vi "get_transitionTrigger.vi"(0 "NInstrSim_DFSMVisitor":refnum<class "NInstrSim_DFSMVisitor.lvclass">, 5 "error in (no error)":errorcluster) -> (14 "NInstrSim_DFSMVisitor":refnum<class "NInstrSim_DFSMVisitor.lvclass">, 16 "Trigger":T1, 17 "deviceVisitor":refnum<class "HGF_DeviceVisitor.lvclass">, 19 "error out":errorcluster)   [LabVIEW 2009, in "HGF_DIM_DFSM_Examples.lvlib" / "NInstrSim_DFSMVisitor.lvclass"]
doc: "This VI returns the HGF_DeviceFSM.lvsc transition trigger and device visitor."
uses:
  NInstrSim_DFSMVisitor.lvclass
  lib.lib/HGF_LVC/HGF_StateCharts/HGF_DeviceFSM/HGF_DeviceFSM.lvsc/Trigger.ctl
  lib.lib/HGF_LVC/HGF_DeviceBaseClasses/HGF_DeviceVisitor/HGF_DeviceVisitor.lvclass
  NInstrSim_ConfigureWaveformType/NInstrSim_ConfigureWaveformType.lvclass
  lib.lib/HGF_LVC/HGF_StateCharts/HGF_DFSMVisitor/HGF_DFSMVisitor.lvclass
  lib.lib/HGF_LVC/HGF_BaseClasses/HGF_NetworkVisitor/HGF_NetworkVisitor.lvclass
  lib.lib/HGF_LVC/HGF_StateCharts/HGF_DeviceFSM/HGF_DeviceFSM.lvsc
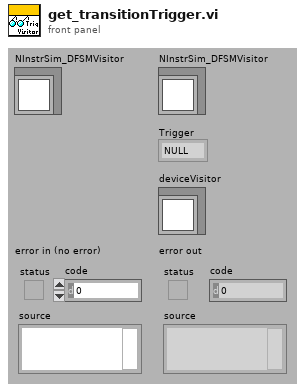
[diagram p1: front panel]
types:
  T1 = typedef "HGF_DeviceFSM.lvlib/HGF_DeviceFSM.lvsc/Trigger.ctl" = enum16{"NULL", "configure", "fault", "error", "resetError", "STOP", "visit", "not_configured", "done", "ok", "previsit", "configured"}
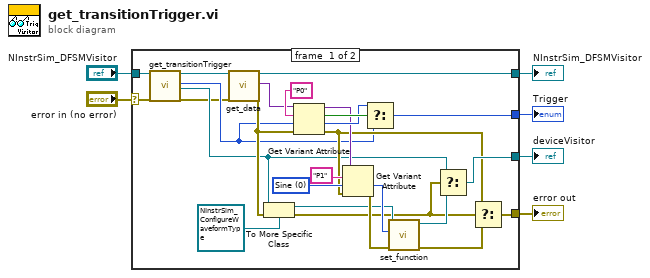
[diagram p0: block diagram]
diagram:
  n1 = case shown="No Error" "error in (no error)" {
    selector: "error in (no error)" -> [w7 w33]
    tunnel: [w13 w33] -> w1
    tunnel: [w30 w34] -> w4
    tunnel: "NInstrSim_DFSMVisitor" -> [w12 w34]
    tunnel: [w27 _] -> w3
    tunnel: [w24 _] -> w2
    frame #0 {
      w21 = u16 0 items=["Sine", "Square", "Sine+Noise", "Random", "Chirp"] ("function (0:Sine)")
      n2 = call-parent "get_transitionTrigger.vi"("HGF_DFSMVisitor"=w12, "error in (no error)"=w7) -> ("HGF_DFSMVisitor"=w11:refnum<class "NInstrSim_DFSMVisitor.lvclass">, "Trigger"=w10:T1, "deviceVisitor"=w9:refnum<class "HGF_DeviceVisitor.lvclass">, "error out"=w8:errorcluster)  [unwired: 14 in]
      n3 = call "get_data.vi"("HGF_NetworkData"=w11, "error in (no error)"=w8) -> ("dup HGF_NetworkData"=w30:refnum<class "NInstrSim_DFSMVisitor.lvclass">, "data"=w31:variant, "error out"=w25:errorcluster)  [unwired: 15 out]
      n4 = To More Specific Class(target class=refnum<class "NInstrSim_ConfigureWaveformType.lvclass"> refnum ("HB_HGF_Test.lvlib:NInstrSim_ConfigureWaveformType.lvclass"), reference=w9, error in=w25) -> (specific class reference=w18:refnum<class "NInstrSim_ConfigureWaveformType.lvclass">, error out=w16:errorcluster)
      n5 = Get Variant Attribute(Variant=w31, name="P0", default value (empty Variant)=w10, error in=w25) -> (duplicate Variant=w22:variant, found=w29:bool, value=w28:T1, error out=w15:errorcluster)
      n6 = Get Variant Attribute(Variant=w22, name="P1", default value (empty Variant)=w21, error in=w15) -> (value=w19:u16, error out=w20:errorcluster)  [unwired: 2 out]
      n7 = Select(t=w28, s=w29, f=w10) -> (s? t:f=w27:T1)
      n8 = call "set_function.vi"("error in (no error)"=w20, "function (0:Sine)"=w19, "NInstrSim_ConfigureWaveformType"=w18) -> ("error out"=w14:errorcluster, "dup NInstrSim_ConfigureWaveformType"=w17:refnum<class "NInstrSim_ConfigureWaveformType.lvclass">)  [unwired: 7 out]
      n9 = Select(t=w9, s=w16, f=w17) -> (s? t:f=w24:refnum<class "HGF_DeviceVisitor.lvclass">)
      n10 = Select(t=w15, s=w16, f=w14) -> (s? t:f=w13:errorcluster)
    }
    frame #1 {
    }
  }
  "error out" <- w1
  "NInstrSim_DFSMVisitor" <- w4
  "Trigger" <- w3
  "deviceVisitor" <- w2
